vi "update_sampling_mode.vi"(8 "error in (no error)":errorcluster, 11 "DAQmxWriteSignals in":refnum<class "SignalWriterDL090202DAQmx.lvclass">) -> (0 "error out":errorcluster, 3 "DAQmxWriteSignals out":refnum<class "SignalWriterDL090202DAQmx.lvclass">)   [LabVIEW 2010, in "SignalWriterDL090202DAQmx.lvclass"]
uses:
  SignalWriterDL090202DAQmx.lvclass
  <vilib>/DAQmx/configure/timing.llb/DAQmx Timing (Sample Clock).vi
  <vilib>/DAQmx/configure/trigger.llb/DAQmx Start Trigger (None).vi
  <vilib>/DAQmx/configure/trigger.llb/DAQmx Start Trigger (Digital Edge).vi
  Program Files/National Instruments/LabVIEW 2010/resource/objmgr/daqmx.rc
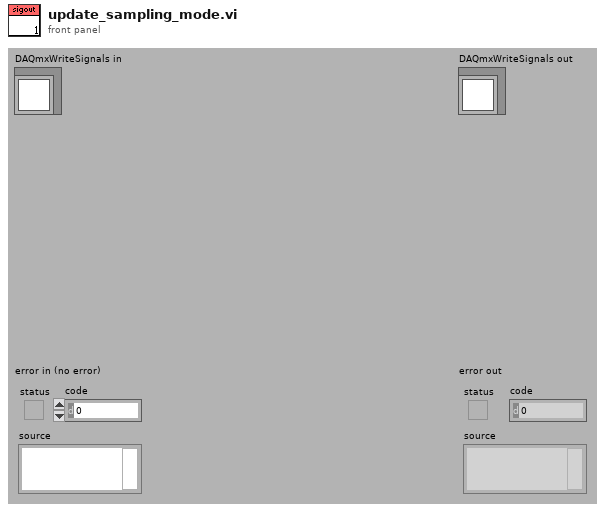
[diagram p1: front panel]
types:
  T1 = typedef "SignalWriterDL090202DAQmx.lvclass/trigger_edge_enum.ctl" = enum16{"rising", "falling"}
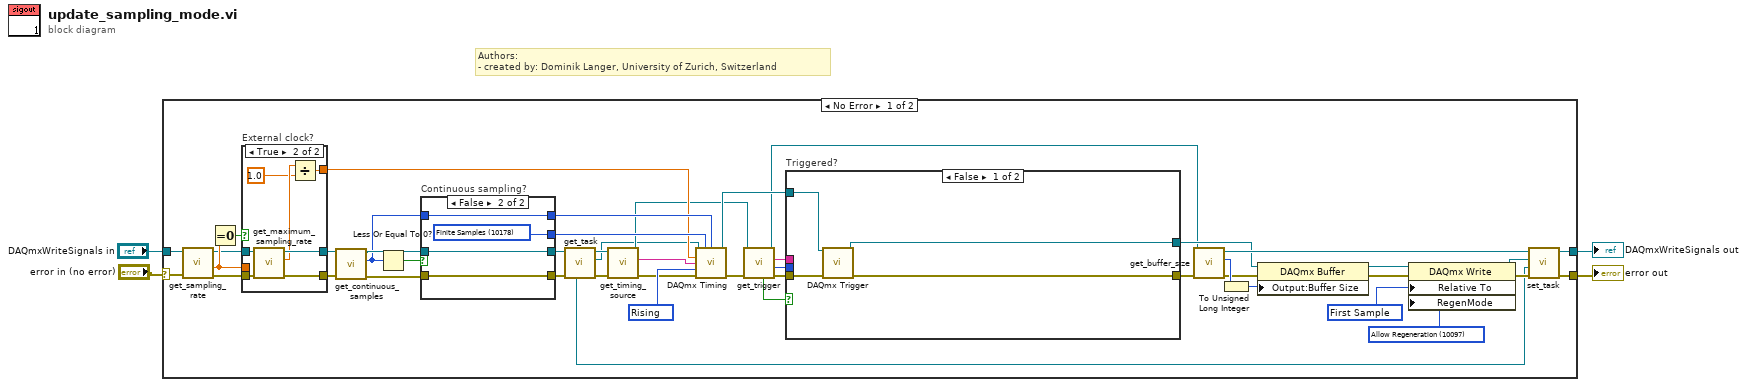
[diagram p0: block diagram]
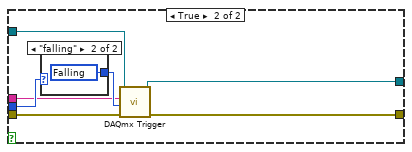
[diagram p2: hidden frame]
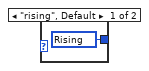
[diagram p3: hidden frame]
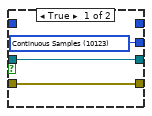
[diagram p4: hidden frame]
diagram:
  # "Authors: \n- created by: Dominik Langer, University of Zurich, Switzerland"
  n1 = case shown="No Error" "error in (no error)" {
    selector: "error in (no error)" -> [w26 w82]
    tunnel: [w18 w82] -> w3
    tunnel: [w17 w81] -> w2
    tunnel: "DAQmxWriteSignals in" -> [w25 w81]
    frame No Error {
      w46 = 10280 items=["Rising"=10280, "Falling"=10171] ("active edge")
      w35 = 10097 items=["Allow Regeneration"=10097, "Do Not Allow Regeneration"=10158] ("RegenMode")
      w27 = 10424 items=["First Sample"=10424, "Current Write Position"=10430] ("RelativeTo")
      n2 = call-dynamic "get_sampling_rate.vi"("error in (no error)"=w26, "GenericWriteSignals in"=w25) -> ("error out"=w37:errorcluster, "sampling rate (Hz)"=w40:dbl, "GenericWriteSignals out"=w38:refnum<class "SignalWriterDL090202DAQmx.lvclass">)  [unwired: 7 out]
      n3 = Equal To 0?(x=w40) -> (x = 0?=w39:bool)
      n4 = case "External clock?" shown="True" w39 {
        tunnel: [w72 w80] -> w48
        tunnel: [w73 w79] -> w47
        tunnel: [w71 w77] -> w41
        tunnel: w37 -> [w73 w75]
        tunnel: w38 -> [w72 w74]
        tunnel: w40 -> [w71 _]
        frame False {
        }
        frame True {
          n5 = call-dynamic "get_maximum_sampling_rate.vi"("error in (no error)"=w75, "DAQmxWriteSignals.lvclass in"=w74) -> ("error out"=w79:errorcluster, "maximum sampling rate"=w78:dbl[unit], "DAQmxWriteSignals.lvclass out"=w80:refnum<class "SignalWriterDL090202DAQmx.lvclass">)  [unwired: 7 out]
          n6 = Divide(x=w78, y=dbl[unit] 1.0) -> (x/y=w77:dbl)
        }
      }
      n7 = call-dynamic "get_continuous_samples.vi"("error in (no error)"=w47, "GenericWriteSignals.lvclass in"=w48) -> ("error out"=w50:errorcluster, "continuous samples"=w19:i32, "GenericWriteSignals.lvclass out"=w49:refnum<class "SignalWriterDL090202DAQmx.lvclass">)  [unwired: 7 out]
      n8 = Less Or Equal To 0?(x=w19) -> (x <= 0?=w20:bool)
      n9 = case "Continuous sampling?" shown="False" w20 {
        tunnel: [w65 w69] -> w24
        tunnel: [w64 w68] -> w23
        tunnel: w50 -> [w65 w69]
        tunnel: w49 -> [w64 w68]
        tunnel: [w66 w70] -> w44
        tunnel: [_ w67] -> w45
        tunnel: w19 -> [_ w67]
        frame True {
          w66 = 10123 items=["Finite Samples"=10178, "Continuous Samples"=10123, "Hardware Timed Single Point"=12522] ("sample mode")
        }
        frame False {
          w70 = 10178 items=["Finite Samples"=10178, "Continuous Samples"=10123, "Hardware Timed Single Point"=12522] ("sample mode")
        }
      }
      n10 = call-dynamic "get_task.vi"("error in (no error)"=w24, "DAQmxWriteSignals in"=w23) -> ("error out"=w21:errorcluster, "writer task"=w6:refnum<k21>, "DAQmxWriteSignals out"=w22:refnum<class "SignalWriterDL090202DAQmx.lvclass">, "counter task"=w5:refnum<k21>)  [unwired: 6 out]
      n11 = call-dynamic "get_timing_source.vi"("error in (no error)"=w21, "DAQmxWriteSignals.lvclass in"=w22) -> ("error out"=w43:errorcluster, "timing source"=w42:tag, "DAQmxWriteSignals.lvclass out"=w10:refnum<class "SignalWriterDL090202DAQmx.lvclass">)  [unwired: 7 out]
      n12 = call-poly <vilib>:"DAQmx Timing.vi"("task/channels in"=w6, "sample mode"=w44, "samples per channel"=w45, "rate"=w41, "source"=w42, "active edge"=w46, "error in"=w43) -> ("task out"=w16:refnum<k21>, "error out"=w13:errorcluster)  [unwired: 7 out]
      n13 = call-dynamic "get_trigger.vi"("error in (no error)"=w13, "DAQmxWriteSignals in"=w10) -> ("error out"=w12:errorcluster, "edge"=w9:T1, "digital trigger line"=w8:tag, "DAQmxWriteSignals out"=w7:refnum<class "SignalWriterDL090202DAQmx.lvclass">, "trigger set?"=w11:bool)  [unwired: 5 out]
      n14 = case "Triggered?" shown="False" w11 {
        tunnel: w16 -> [w51 w61]
        tunnel: [w52 w55] -> w15
        tunnel: w12 -> [w54 w60]
        tunnel: [w53 w56] -> w14
        tunnel: w9 -> [_ w58]
        tunnel: w8 -> [_ w57]
        frame False {
          n15 = call-poly <vilib>:"DAQmx Trigger.vi"("task/channels in"=w51, "error in"=w54) -> ("task out"=w52:refnum<k21>, "error out"=w53:errorcluster)  [unwired: 12 out]
        }
        frame True {
          n16 = case shown="\"falling\"" w58 {
            tunnel: [w62 w63] -> w59
            frame "rising", Default {
              w62 = 10280 items=["Rising"=10280, "Falling"=10171] ("edge")
            }
            frame "falling" {
              w63 = 10171 items=["Rising"=10280, "Falling"=10171] ("edge")
            }
          }
          n17 = call-poly <vilib>:"DAQmx Trigger.vi"("task/channels in"=w61, "source"=w57, "edge"=w59, "error in"=w60) -> ("task out"=w55:refnum<k21>, "error out"=w56:errorcluster)  [unwired: 10 out]
        }
      }
      n18 = call-dynamic "get_buffer_size.vi"("error in (no error)"=w14, "GenericWriteSignals.lvclass in"=w7) -> ("error out"=w31:errorcluster, "buffer size (samples)"=w33:i32, "GenericWriteSignals.lvclass out"=w32:refnum<class "SignalWriterDL090202DAQmx.lvclass">)  [unwired: 7 out]
      n19 = To Unsigned Long Integer(number=w33) -> (unsigned 32bit integer=w34:u32)
      n20 = property class="DAQmx Buffer"(reference=w15, error in=w31, "Output:Buffer Size"=w34) -> (reference out=w36:refnum<k21>, error out=w28:errorcluster)
      n21 = property class="DAQmx Write"(reference=w36, error in=w28, "Relative To"=w27, "RegenMode"=w35) -> (reference out=w30:refnum<k21>, error out=w29:errorcluster)
      n22 = call-dynamic "set_task.vi"("error in (no error)"=w29, "counter task"=w5, "output task"=w30, "DAQmxWriteSignals in"=w32) -> ("error out"=w18:errorcluster, "DAQmxWriteSignals out"=w17:refnum<class "SignalWriterDL090202DAQmx.lvclass">)  [unwired: 6 out]
    }
    frame Error {
    }
  }
  "error out" <- w3
  "DAQmxWriteSignals out" <- w2
